vi "Translation Stage Coarse.vi"(8 "error in (no error)":errorcluster, 10 "Translation Stages.lvclass":refnum<class "Translation Stages.lvclass">, 11 "Translation Stage Coarse In":refnum<class "Translation Stage Coarse.lvclass">) -> (0 "error out":errorcluster, 3 "Translation Stage Coarse Out":refnum<class "Translation Stage Coarse.lvclass">)   [LabVIEW 2015, in "Translation Stage Coarse.lvclass"]
uses:
  Translation Stage Coarse.lvclass
  Instruments/Translation Stages/Translation Stages.lvclass
  Scanner/Scanner.lvclass
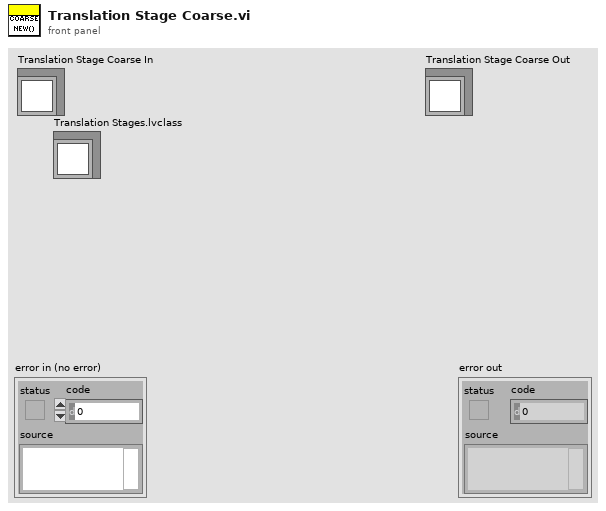
[diagram p1: front panel]
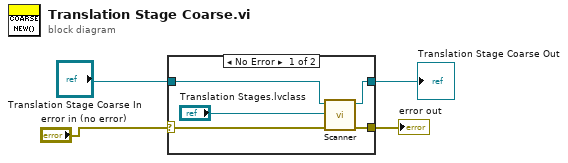
[diagram p0: block diagram]
diagram:
  n1 = case shown="No Error" "error in (no error)" {
    selector: "error in (no error)" -> [w7 w11]
    tunnel: [w6 w11] -> w3
    tunnel: [w9 w10] -> w1
    tunnel: "Translation Stage Coarse In" -> [w8 w10]
    frame No Error {
      n2 = call "Scanner.vi"("error in (no error)"=w7, "Scannable"="Translation Stages.lvclass", "Scanner.lvclass in"=w8) -> ("error out"=w6:errorcluster, "Scanner.lvclass out"=w9:refnum<class "Translation Stage Coarse.lvclass">)  [unwired: 1 in, 6 out]
    }
    frame Error {
    }
  }
  "error out" <- w3
  "Translation Stage Coarse Out" <- w1
